vi "Teleop.vi"(10 "Match Info":T1={"Autonomous Elapsed Seconds"=0.0, "TeleOp Elapsed Seconds"=0.0, "Disabled Elapsed Seconds"=0.0, "Visited Autonomous"=FALSE, "Visited TeleOp"=FALSE, "Visited Disabled"=FALSE, "Autonomous Settings"={"Autonomous Style"=enum."Independent", "VI Refnum"=refnum}}, 11 "Call Context":T2) -> ()   [LabVIEW 2013]
doc: "This VI is called for each TeleOp packet received from the DS where the robot is not disabled. It is often used to read from the joysticks and update I/O or to update setpoints for timed control loops. It should complete and return within 20 milliseconds or it may miss DS packets."
uses:
  <vilib>/Rock Robotics/WPI/DriverStation/WPI_DriverStationDerivedRobotMode.ctl
  <vilib>/Rock Robotics/WPI/DriverStation/WPI_DriverStationMatch Info.ctl
  TeleopInstruction.ctl
  Robot Global Data.vi
  <vilib>/Rock Robotics/WPI/Joystick/WPI_JoystickGetSetRefNum.vi
panel:
  out "Time":u32
  in  "Xbox?":bool
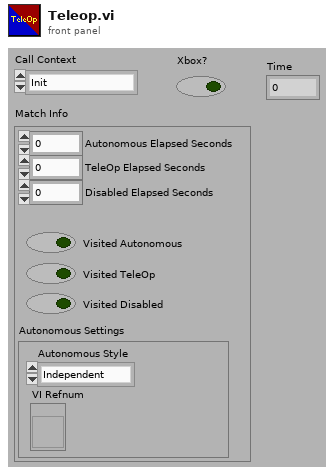
[diagram p1: front panel]
types:
  T1 = typedef "WPI_DriverStationMatch Info.ctl" = cluster{"Autonomous Elapsed Seconds":dbl, "TeleOp Elapsed Seconds":dbl, "Disabled Elapsed Seconds":dbl, "Visited Autonomous":bool, "Visited TeleOp":bool, "Visited Disabled":bool, "Autonomous Settings":cluster{"Autonomous Style":enum16{"Iterative", "Independent"}, "VI Refnum":refnum<vi>}}
  T2 = typedef "WPI_DriverStationDerivedRobotMode.ctl" = enum16{"Init", "Execute", "Stop"}
  T3 = typedef "TeleopInstruction.ctl" = cluster{"cDriveLeft":dbl, "cDriveRight":dbl, "cAutoDistance":bool, "cHalfDrive":bool, "cStraightDrive":bool, "cReverseDrive":bool, "cSonicShifter":bool, "cRoller":dbl, "cCollector":dbl, "cServo":dbl, "cPass":bool, "cCatch":bool, "cCollectorWrap":bool, "cShooter":bool, "cClapperIn":bool, "cClapperOut":bool, "cFiringPneumatic":bool, "cKickerPneumatic":bool, "cRollerPneumatic":bool, "TeleopID":i32}
  T4 = typedef "WPI_JoystickDevRef.ctl" = cluster{"Device":T5}
  T5 = typedef "WPI_JoystickDeviceEnum.ctl" = enum16{"USB 1", "USB 2", "USB 3", "USB 4", "Kinect 1", "Kinect 2"}
  T6 = typedef "WPI_JoystickButtonState.ctl" = cluster{"Button 1":bool, "Button 2":bool, "Button 3":bool, "Button 4":bool, "Button 5":bool, "Button 6":bool, "Button 7":bool, "Button 8":bool, "Button 9":bool, "Button 10":bool, "Button 11":bool, "Button 12":bool}
  T7 = cluster{"axis 1 (x)":dbl, "axis 2 (y)":dbl, "axis 3 (throttle)":dbl, "axis 4":dbl, "axis 5":dbl, "axis 6":dbl}
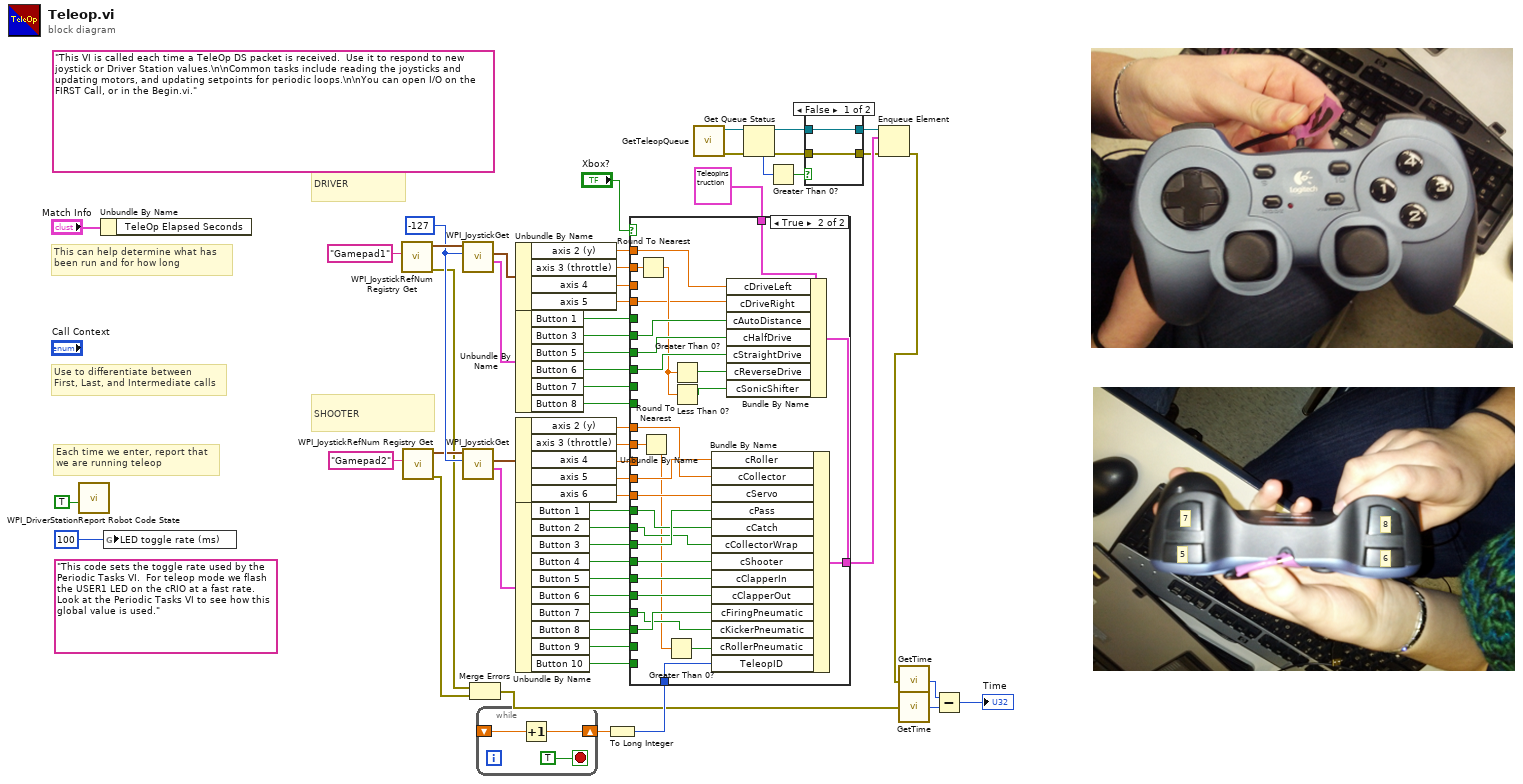
[diagram p0: block diagram]
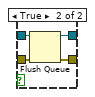
[diagram p2: hidden frame]
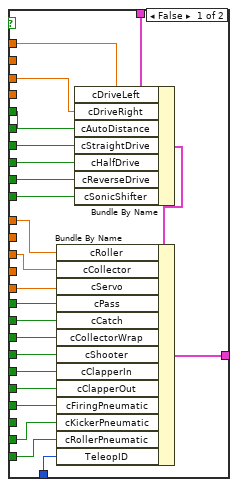
[diagram p3: hidden frame]
diagram:
  w50 = i8 -127 ("Scaler")
  (unwired) "This code sets the toggle rate used by the Periodic Tasks VI.  For teleop mode we flash the USER1 LED on the cRIO at a fast rate.  Look at the Periodic Tasks VI to see how this global value is used."
  (unwired) "This VI is called each time a TeleOp DS packet is received.  Use it to respond to new joystick or Driver Station values.\n\nCommon tasks include reading the joysticks and updating motors, and updating setpoints for periodic loops.\n\nYou can open I/O on the FIRST Call, or in the Begin.vi."
  # "SHOOTER"
  # "DRIVER"
  # "5"
  # "7"
  # "6"
  # "8"
  # "Each time we enter, report that\nwe are running teleop"
  # "Use to differentiate between\nFirst, Last, and Intermediate calls"
  # "This can help determine what has\nbeen run and for how long"
  n1 = call <vilib>:"WPI_DriverStationReport Robot Code State.vi"("TeleOp"=TRUE ("Autonomous")) -> ()  [unwired: 10 in, 1 out]
  n2 = Unbundle By Name("Match Info") -> ()  [unwired: 1 out]
  n3 = global write "Robot Global Data.vi" "LED toggle rate (ms)"(u32 100 ("LED ms toggle rate")) -> ()
  n4 = call <vilib>:"WPI_JoystickRefNum Registry Get.vi"("refnum name"="Gamepad1") -> ("error out"=w14:errorcluster, "JoystickDevRef"=w51:T4)  [unwired: 9 in]
  n5 = call <vilib>:"WPI_JoystickRefNum Registry Get.vi"("refnum name"="Gamepad2") -> ("error out"=w15:errorcluster, "JoystickDevRef"=w49:T4)  [unwired: 9 in]
  n6 = call <vilib>:"WPI_JoystickGet.vi"("Scaler"=w50, "JoystickDevRef"=w51) -> ("Buttons"=w47:T6, "Axes"=w48:T7)  [unwired: 3 in, 1 out]
  n7 = call <vilib>:"WPI_JoystickGet.vi"("Scaler"=w50, "JoystickDevRef"=w49) -> ("Buttons"=w45:T6, "Axes"=w46:T7)  [unwired: 3 in, 1 out]
  n8 = Merge Errors(w14, w15) -> (w13:errorcluster)
  n9 = while {
    shift-right: [w59] -> w30
    shift-left: _ -> [w58]
    stop <- TRUE stop-if-true
    n10 = Increment(x=w58) -> (x+1=w59:dbl)
  }
  n11 = Unbundle By Name(w48) -> ("axis 2 (y)"=w19:dbl, "axis 3 (throttle)"=w17:dbl, "axis 4"=w18:dbl, "axis 5"=w16:dbl)
  n12 = Unbundle By Name(w47) -> ("Button 1"=w31:bool, "Button 3"=w32:bool, "Button 5"=w21:bool, "Button 6"=w43:bool, "Button 7"=w42:bool, "Button 8"=w41:bool)
  n13 = Unbundle By Name(w46) -> ("axis 2 (y)"=w35:dbl, "axis 3 (throttle)"=w36:dbl, "axis 5"=w22:dbl, "axis 6"=w23:dbl)  [unwired: 1 out]
  n14 = Unbundle By Name(w45) -> ("Button 1"=w28:bool, "Button 2"=w29:bool, "Button 3"=w33:bool, "Button 4"=w34:bool, "Button 5"=w37:bool, "Button 6"=w40:bool, "Button 7"=w39:bool, "Button 8"=w38:bool, "Button 9"=w26:bool, "Button 10"=w24:bool)
  n15 = To Long Integer(number=w30) -> (32bit integer=w27:i32)
  n16 = case shown="True" "Xbox?" {
    tunnel: T3 {"cDriveLeft"=0.0, "cDriveRight"=0.0, "cAutoDistance"=FALSE, "cHalfDrive"=FALSE, "cStraightDrive"=FALSE, "cReverseDrive"=FALSE, "cSonicShifter"=FALSE, "cRoller"=0.0, "cCollector"=0.0, "cServo"=0.0, "cPass"=FALSE, "cCatch"=FALSE, "cCollectorWrap"=FALSE, "cShooter"=FALSE, "cClapperIn"=FALSE, "cClapperOut"=FALSE, "cFiringPneumatic"=FALSE, "cKickerPneumatic"=FALSE, "cRollerPneumatic"=FALSE, "TeleopID"=0} ("TeleopInstruction") -> [w82 w108]
    tunnel: w18 -> [w61 _]
    tunnel: w43 -> [w81 w104]
    tunnel: w42 -> [w80 _]
    tunnel: w41 -> [w79 _]
    tunnel: w40 -> [w66 w90]
    tunnel: w39 -> [w65 w88]
    tunnel: w38 -> [_ w89]
    tunnel: w37 -> [w67 w91]
    tunnel: w36 -> [_ w99]
    tunnel: w35 -> [w74 w97]
    tunnel: w34 -> [w68 w92]
    tunnel: w33 -> [w69 w95]
    tunnel: w32 -> [_ w106]
    tunnel: w31 -> [w78 _]
    tunnel: w29 -> [w70 w93]
    tunnel: w28 -> [w71 w94]
    tunnel: w22 -> [w73 _]
    tunnel: w27 -> [w62 w85]
    tunnel: w26 -> [w64 _]
    tunnel: w24 -> [w63 _]
    tunnel: w23 -> [w72 w96]
    tunnel: w22 -> [_ w98]
    tunnel: w21 -> [w77 w105]
    tunnel: [w75 w100] -> w20
    tunnel: w19 -> [w60 w107]
    tunnel: w17 -> [_ w84]
    tunnel: w16 -> [_ w83]
    frame False {
      n17 = Bundle By Name(cluster=w82, "cDriveLeft"=w60, "cDriveRight"=w61, "cAutoDistance"=w78, "cStraightDrive"=w77, "cHalfDrive"=w81, "cReverseDrive"=w80, "cSonicShifter"=w79) -> (w76:T3)
      n18 = Bundle By Name(cluster=w76, "cRoller"=w74, "cCollector"=w73, "cServo"=w72, "cPass"=w71, "cCatch"=w70, "cCollectorWrap"=w69, "cShooter"=w68, "cClapperIn"=w67, "cClapperOut"=w66, "cFiringPneumatic"=w65, "cKickerPneumatic"=w64, "cRollerPneumatic"=w63, "TeleopID"=w62) -> (w75:T3)
    }
    frame True {
      n19 = Round To Nearest(number=w84) -> (nearest integer value=w101:dbl)
      n20 = Round To Nearest(number=w99) -> (nearest integer value=w87:dbl)
      n21 = Greater Than 0?(x=w87) -> (x > 0?=w86:bool)
      n22 = Greater Than 0?(x=w101) -> (x > 0?=w102:bool)
      n23 = Less Than 0?(x=w101) -> (x < 0?=w103:bool)
      n24 = Bundle By Name(cluster=w108, "cDriveLeft"=w107, "cDriveRight"=w83, "cAutoDistance"=w106, "cHalfDrive"=w105, "cStraightDrive"=w104, "cReverseDrive"=w102, "cSonicShifter"=w103) -> (w100:T3)
      n25 = Bundle By Name(cluster=w100, "cRoller"=w98, "cCollector"=w97, "cServo"=w96, "cPass"=w95, "cCatch"=w94, "cCollectorWrap"=w93, "cShooter"=w92, "cClapperIn"=w91, "cClapperOut"=w90, "cFiringPneumatic"=w89, "cKickerPneumatic"=w88, "cRollerPneumatic"=w86, "TeleopID"=w85) -> ()  [unwired: 1 out]
    }
  }
  n26 = call "GetTeleopQueue.vi"() -> ("error out"=w7:errorcluster, "queue out"=w8:refnum<queue>)  [unwired: 10 in]
  n27 = Get Queue Status(queue=w8, error in (no error)=w7) -> (queue out=w5:refnum<queue>, error out=w4:errorcluster, # elements in queue=w6:i32)  [unwired: 1 in, 5 out]
  n28 = Greater Than 0?(x=w6) -> (x > 0?=w3:bool)
  n29 = case shown="False" w3 {
    tunnel: w5 -> [w110 w114]
    tunnel: w4 -> [w109 w113]
    tunnel: [w110 w112] -> w2
    tunnel: [w109 w111] -> w1
    frame False {
    }
    frame True {
      n30 = Flush Queue(queue=w114, error in (no error)=w113) -> (queue out=w112:refnum<queue>, error out=w111:errorcluster)  [unwired: 1 out]
    }
  }
  n31 = Enqueue Element(queue=w2, element=w20, error in (no error)=w1) -> (error out=w10:errorcluster)  [unwired: 1 in, 2 out]
  n32 = call "GetTime.vi"("error in"=w10) -> ("Time"=w9:u32)
  n33 = call "GetTime.vi"("error in"=w13) -> ("Time"=w12:u32)
  n34 = Subtract(x=w9, y=w12) -> (x-y=→"Time":u32)
